vi "Read Command Status.vi"(8 "error in (no error)":errorcluster, 11 "Receiver Command in":refnum<class "Receiver Command.lvclass">) -> (0 "error out":errorcluster, 2 "Command Status":T1, 3 "Receiver Command out":refnum<class "Receiver Command.lvclass">)   [LabVIEW 2013, in "Receiver.lvlib" / "Receiver Commands Using Processor.lvlib" / "Receiver Command.lvclass"]
uses:
  Receiver Command.lvclass
  Command Processor/Command/Command Status.ctl
  Command Processor/Command/State Status.ctl
  Command Processor/Command/Command.lvclass
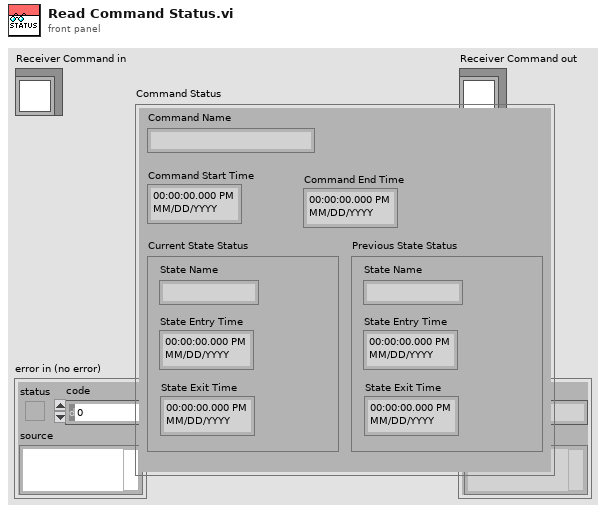
[diagram p1: front panel]
types:
  T1 = typedef "Command Processor.lvlib/Command.lvlib/Command.lvclass/Command Status.ctl" = cluster{"Command Name":string, "Current State Status":T2, "Command Start Time":timestamp, "Command End Time":timestamp, "Previous State Status":T2}
  T2 = typedef "Command Processor.lvlib/Command.lvlib/Command.lvclass/State Status.ctl" = cluster{"State Name":string, "State Entry Time":timestamp, "State Exit Time":timestamp}
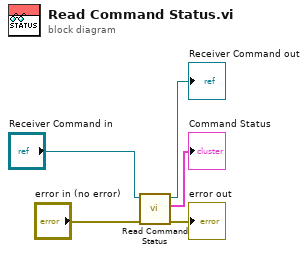
[diagram p0: block diagram]
diagram:
  n1 = call-parent "Read Command Status.vi"("error in (no error)"="error in (no error)", "Command in"="Receiver Command in") -> ("error out"=→"error out":errorcluster, "Command Status"=→"Command Status":T1, "Command out"=→"Receiver Command out":refnum<class "Receiver Command.lvclass">)  [unwired: 7 in]
